vi "toml_api_remove.vi"(7 "resolved path":path, 8 "error in (no error)":errorcluster, 9 "key":string, 10 "section":string, 11 "vi in":refnum<vi>) -> (0 "error out":errorcluster, 2 "key exists":bool, 3 "vi out":refnum<vi>)   [LabVIEW 2017]
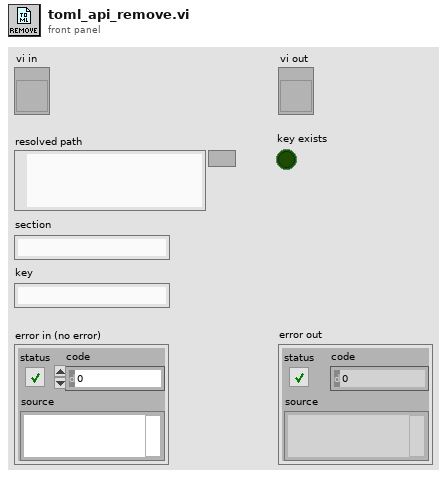
[diagram p1: front panel]
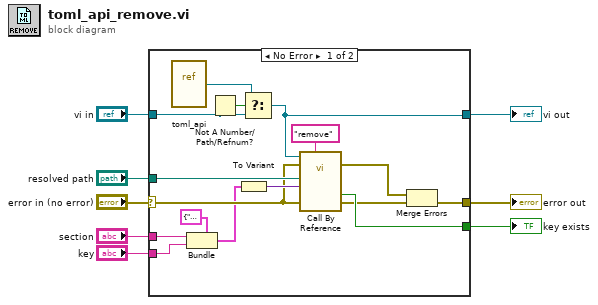
[diagram p0: block diagram]
diagram:
  n1 = case shown="No Error" "error in (no error)" {
    selector: "error in (no error)" -> [w15 w26]
    tunnel: [w23 _] -> w8
    tunnel: "resolved path" -> [w21 _]
    tunnel: [w17 w26] -> w6
    tunnel: "vi in" -> [w14 w25]
    tunnel: [w13 w25] -> w3
    tunnel: "section" -> [w12 _]
    tunnel: "key" -> [w11 _]
    frame No Error {
      n2 = vi-ref "toml_api.vi"() -> (w20:refnum<vi>)
      n3 = Bundle(cluster=cluster{"section":string, "key":string} {"section"="", "key"=""}, "section"=w12, "key"=w11) -> (w10:cluster{"section":string, "key":string})
      n4 = Not A Number/Path/Refnum?(number/path/refnum=w14) -> (NaN/Path/Refnum?=w19:bool)
      n5 = To Variant(anything=w10) -> (Variant=w24:variant)
      n6 = Select(t=w20, s=w19, f=w14) -> (s? t:f=w13:refnum<vi>)
      n7 = call-by-ref "?"(reference=w13, error in=w15, "cmd"="remove", 8:"error in (no error)"=w15, "data in"=w24, "path in"=w21) -> (error out=w16:errorcluster, 0:"error out"=w22:errorcluster, "return"=w23:bool)  [unwired: 4 in, 3 out]
      n8 = Merge Errors(w16, w22) -> (w17:errorcluster)
    }
    frame Error {
    }
  }
  "key exists" <- w8
  "error out" <- w6
  "vi out" <- w3
